vi "Camera_Focusing_updated.vi"(0 "Image Path":path=path "C:/images/img1.jpeg", 1 "CURRENT MEAN VALUE":refnum<vi>, 2 "error in":errorcluster, 3 "MEAN VALUE MAX":refnum<vi>, 4 "Filter Type":T2(ring)=enum."Differentiation", 5 "Waveform Chart":refnum<vi>, 6 "Ctl Refnum":refnum<vi>, 14 "Pattern Presence":refnum<vi>) -> (11 "Image out":T1(plugin-control), 12 "Result":bool, 13 "Reverse":bool, 15 "Mean Value Max":sgl=4.1535125 format="%.2f", 16 "error out":errorcluster, 17 "Image Dst Out":T1, 18 "Curent Mean Value":sgl=4.1535125 format="%.2f")   [LabVIEW 2019]
uses:
  <vilib>/vision/Image Controls.llb/IMAQ Image.ctl
  <vilib>/vision/NI_Vision_Development_Module.lvlib
panel:
  out "Pattern Presence":bool=TRUE
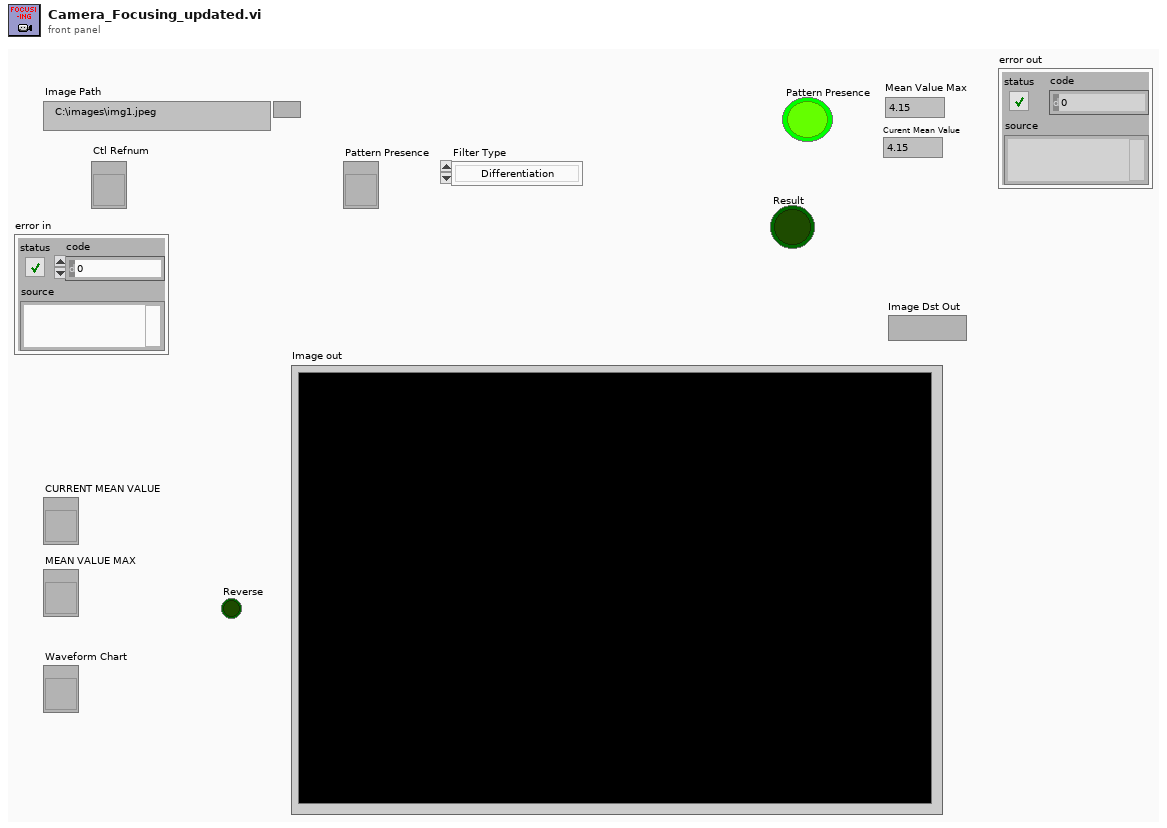
[diagram p1: front panel]
types:
  T1 = typedef "IMAQ Image.ctl" = refnum<image>
  T2 = enum16{"Convolution", "Differentiation", "Gradient", "Prewitt", "Roberts", "Sigma", "Sobel"}
  T3 = enum32{"Differentiation", "Gradient", "Prewitt", "Roberts", "Sigma", "Sobel"}
  T4 = typedef "Image Type" = u32
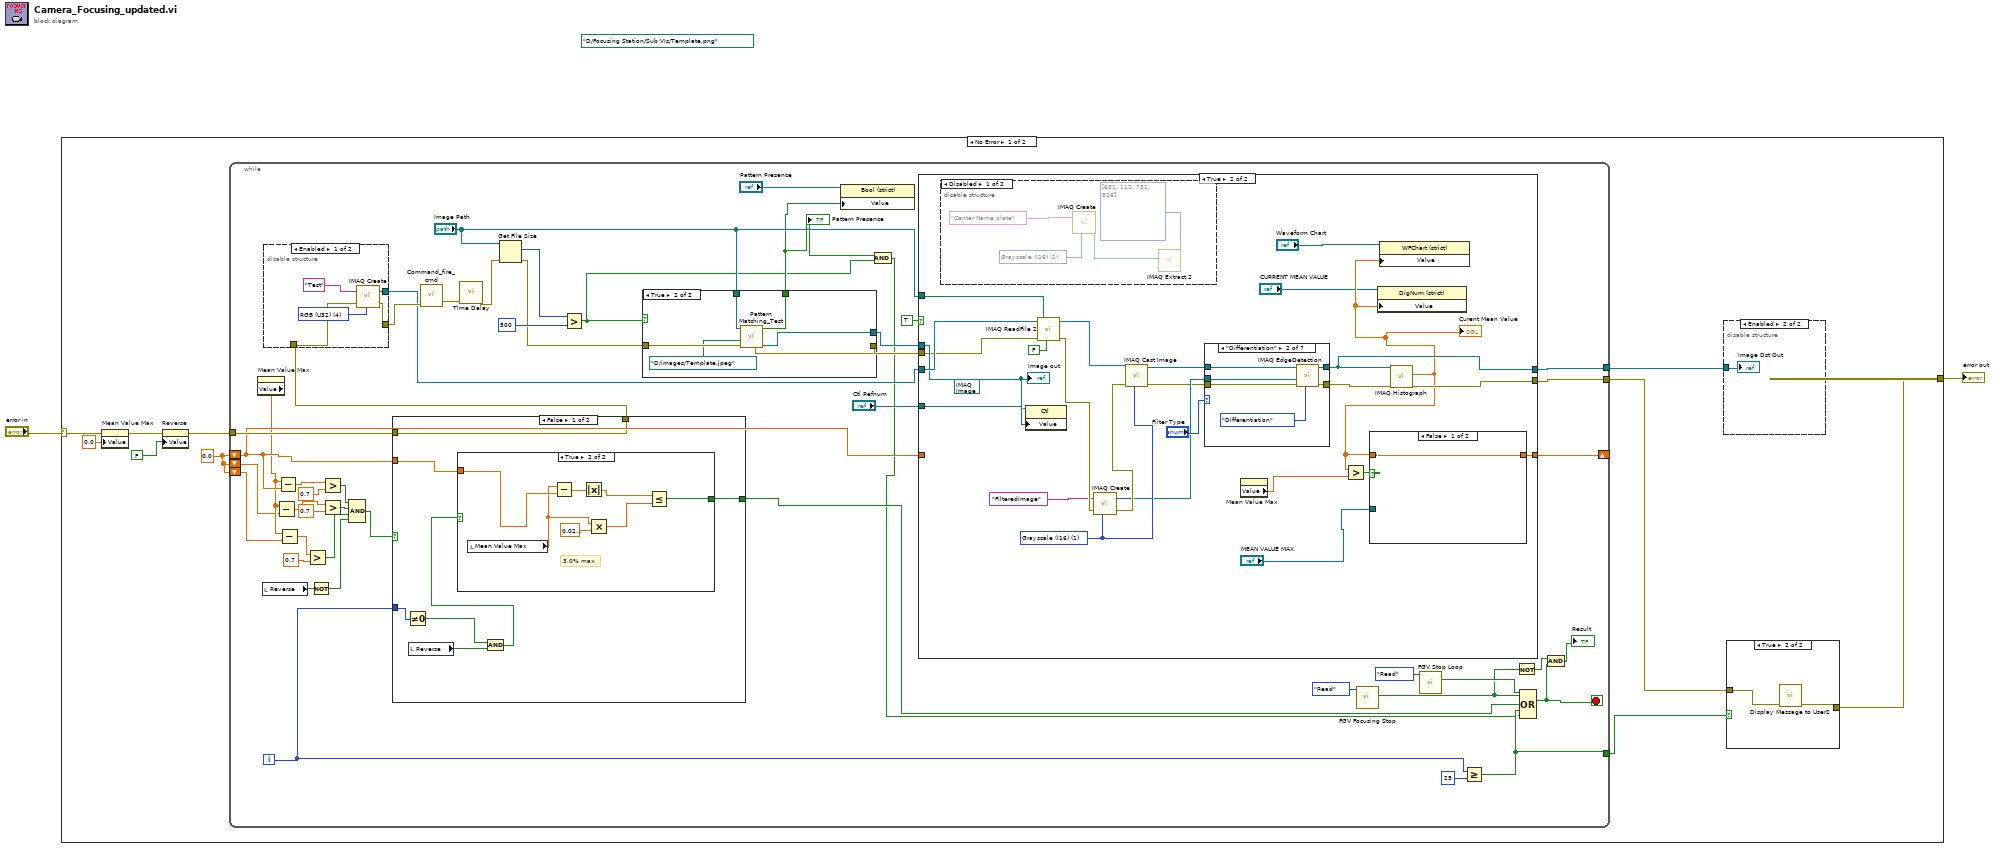
[diagram p0: block diagram]
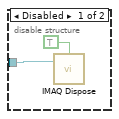
[diagram p3: hidden frame]
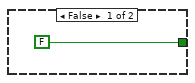
[diagram p6: hidden frame]
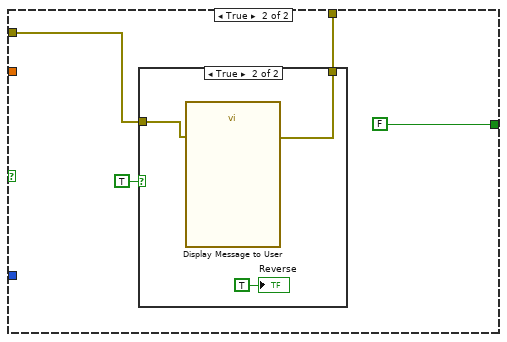
[diagram p7: hidden frame]
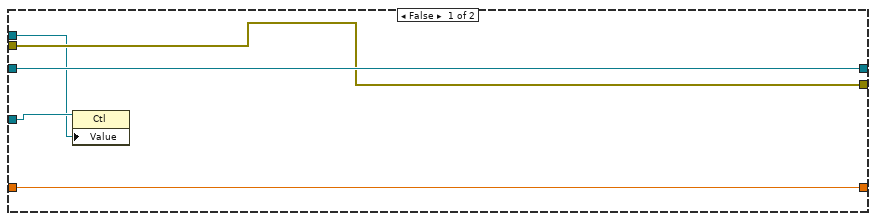
[diagram p9: hidden frame]
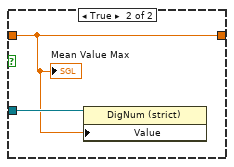
[diagram p11: hidden frame]
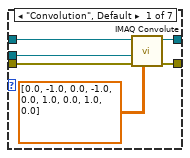
[diagram p12: hidden frame]
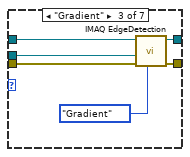
[diagram p13: hidden frame]
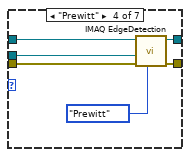
[diagram p14: hidden frame]
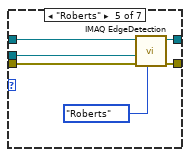
[diagram p15: hidden frame]
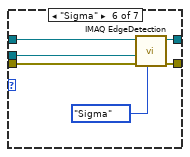
[diagram p16: hidden frame]
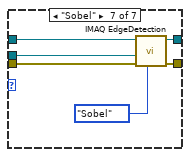
[diagram p17: hidden frame]
diagram:
  (unwired) path "D:/Focusing Station/Sub VIs/Template.png" ("Template file path")
  n1 = case shown="No Error" "error in" {
    selector: "error in" -> [w6 w181]
    tunnel: [w3 w181] -> w2
    frame No Error {
      w9 = 0.0
      n2 = property on="Mean Value Max" class="DigNum (strict)"(error in=w6, "Value"=sgl 0.0 ("Mean Value Max")) -> (error out=w8:errorcluster)  [unwired: 1 in, 1 out]
      n3 = property on="Reverse" class="Bool"(error in=w8, "Value"=FALSE ("Reverse")) -> (error out=w10:errorcluster)  [unwired: 1 in, 1 out]
      n4 = while {
        tunnel: [w66] -> w4
        tunnel: [w65] -> w12
        shift-right: [w57] -> _
        shift-left: w9 -> [w51]
        shift-left: w9 -> [w49]
        shift-left: w9 -> [w48]
        tunnel: w10 -> [w55]
        tunnel: [w30] -> w5
        i -> [w32]
        stop <- w23 stop-if-true
        n5 = property on="Mean Value Max" class="DigNum (strict)"() -> ("Value"=w50:sgl)  [unwired: 2 in, 2 out]
        n6 = local read "Reverse"() -> (w37:bool)
        n7 = Subtract(x=w50, y=w49) -> (x-y=w42:dbl)
        n8 = Subtract(x=w50, y=w51) -> (x-y=w47:dbl)
        n9 = Subtract(x=w50, y=w48) -> (x-y=w43:dbl)
        n10 = Greater?(x=w43, y=0.7) -> (0:w39:bool)
        n11 = Not(x=w37) -> (.not. x?=w36:bool)
        n12 = Greater?(x=w47, y=0.7) -> (0:w41:bool)
        n13 = Greater?(x=w42, y=0.7) -> (0:w40:bool)
        n14 = Compound Arithmetic op=AND(w41, w40, w39, w36) -> (w38:bool)
        n15 = case shown="False" w38 {
          tunnel: w32 -> [w84 _]
          tunnel: [w85 FALSE] -> w34
          tunnel: [w80 w96] -> w56
          tunnel: w55 -> [w80 w95]
          tunnel: w51 -> [w79 _]
          frame False {
            n16 = Not Equal To 0?(x=w84) -> (x != 0?=w82:bool)
            n17 = local read "Reverse"() -> (w83:bool)
            n18 = And(x=w82, y=w83) -> (x .and. y?=w81:bool)
            n19 = case shown="True" w81 {
              tunnel: [FALSE w91] -> w85
              tunnel: w79 -> [_ w88]
              frame False {
              }
              frame True {
                # "3.0% max"
                n20 = local read "Mean Value Max"() -> (w87:sgl)
                n21 = Subtract(x=w87, y=w88) -> (x-y=w93:dbl)
                n22 = Absolute Value(x=w93) -> (abs(x)=w89:dbl)
                n23 = Multiply(x=w87, y=sgl 0.03) -> (x*y=w90:sgl)
                n24 = Less Or Equal?(x=w89, y=w90) -> (x <= y?=w91:bool)
              }
            }
          }
          frame True {
            n25 = case shown="True" TRUE {
              tunnel: [w98 w100] -> w96
              tunnel: w95 -> [w98 w99]
              frame False {
              }
              frame True {
                n26 = call "Display Message to User"("error in (no error)"=w99) -> ("error out"=w100:errorcluster)  [unwired: 9 in, 1 out]
                "Reverse" <- TRUE ("Reverse")
              }
            }
          }
        }
        n27 = disable-structure shown="Enabled" {
          disable-tunnel: [w76 _] -> w61
          disable-tunnel: [w75 _] -> w60
          disable-tunnel: w56 -> [w74 _]
          frame Enabled {
            w77 = T4 4 items=["Grayscale (U8)", "Grayscale (I16)", "Grayscale (SGL)", "Complex (CSG)", "RGB (U32)", "HSL (U32)", "RGB (U64)", "Grayscale (U16)"] ("Image Type")
            n28 = call "IMAQ Create"("Image Name"="Test", "Image Type"=w77, "error in (no error)"=w74) -> ("New Image"=w75:T1, "error out"=w76:errorcluster)  [unwired: 2 in]
          }
          frame Disabled {
          }
        }
        n29 = call "Command_fire_cmd.vi"("error in"=w61) -> ("error out"=w59:errorcluster)  [unwired: 6 in, 2 out]
        n30 = call "Time Delay"("error in (no error)"=w59) -> ("error out"=w33:errorcluster)  [unwired: 10 in]
        n31 = Get File Size(file="Image Path", error in=w33) -> (size (in bytes)=w63:i64, 0:w58:errorcluster)  [unwired: 1 out]
        n32 = Greater?(x=w63, y=i64 500) -> (0:w26:bool)
        n33 = case shown="True" w26 {
          tunnel: "Image Path" -> [_ w73]
          tunnel: w58 -> [w67 w72]
          tunnel: [_ w71] -> w54
          tunnel: [_ w70] -> w27
          tunnel: [w67 w69] -> w53
          frame False {
          }
          frame True {
            n34 = call "Pattern Matching_Test.vi"("error in (no error)"=w72, "Template file path"=path "D:/images/Template.jpeg", "File Path"=w73) -> ("Image out"=w71:T1, "Pattern Presence"=w70:bool, "error out"=w69:errorcluster)  [unwired: 4 in, 2 out]
          }
        }
        "Pattern Presence" <- w27
        n35 = property class="Bool (strict)"(reference="Pattern Presence", "Value"=w27) -> ()  [unwired: 1 in, 2 out]
        n36 = And(x=w27, y=w26) -> (x .and. y?=w19:bool)
        n37 = case shown="True" TRUE {
          tunnel: "Image Path" -> [_ w130]
          tunnel: [w106 w122] -> w57
          tunnel: w51 -> [w106 _]
          tunnel: w60 -> [w105 w121]
          tunnel: [w104 w120] -> w66
          tunnel: [w105 w119] -> w65
          tunnel: w54 -> [w102 w112]
          tunnel: w53 -> [w104 w111]
          tunnel: "Ctl Refnum" -> [w103 w109]
          frame False {
            n38 = property class="Ctl"(reference=w103, "Value"=w102) -> ()  [unwired: 1 in, 2 out]
          }
          frame True {
            (unwired) T1 refnum ("New Image")
            w127 = T4 1 items=["Grayscale (U8)", "Grayscale (I16)", "Grayscale (SGL)", "Complex (CSG)", "RGB (U32)", "HSL (U32)", "RGB (U64)", "Grayscale (U16)"] ("Image Type")
            n39 = disable-structure shown="Disabled" {
              frame Disabled {
                w135 = T4 1 items=["Grayscale (U8)", "Grayscale (I16)", "Grayscale (SGL)", "Complex (CSG)", "RGB (U32)", "HSL (U32)", "RGB (U64)", "Grayscale (U16)"] ("Image Type")
                n40 = call "IMAQ Create"("Image Name"="Center Name plate", "Image Type"=w135) -> ("New Image"=w133:T1)  [unwired: 3 in, 1 out]
                n41 = call "IMAQ Extract 2"("Optional Rectangle"=i32[] [631, 112, 731, 526], "Image Dst"=w133) -> ()  [unwired: 8 in, 2 out]
              }
              frame Enabled {
              }
            }
            n42 = property class="Ctl"(reference=w109, "Value"=w112) -> ()  [unwired: 1 in, 2 out]
            n43 = call "IMAQ ReadFile 2"("Use File Path Image Type"=FALSE, "File Path"=w130, "error in (no error)"=w111, "Image"=w121) -> ("error out"=w129:errorcluster, "Image Out"=w118:T1)  [unwired: 3 in, 3 out]
            n44 = call "IMAQ Create"("Image Name"="FilteredImage", "Image Type"=w127, "error in (no error)"=w129) -> ("New Image"=w125:T1, "error out"=w128:errorcluster)  [unwired: 2 in]
            n45 = call "IMAQ Cast Image"("Image Type"=w127, "error in (no error)"=w128, "Image Src"=w118) -> ("error out"=w108:errorcluster, "Image Dst Out"=w107:T1)  [unwired: 7 in]
            n46 = case shown="\"Differentiation\"" "Filter Type" {
              tunnel: w107 -> [w143 w149 w155 w161 w167 w173 w179]
              tunnel: w108 -> [w142 w148 w154 w160 w166 w172 w178]
              tunnel: w125 -> [w141 w150 w156 w162 w168 w174 w180]
              tunnel: [w140 w145 w151 w157 w163 w169 w175] -> w124
              tunnel: [w139 w146 w152 w158 w164 w170 w176] -> w119
              frame "Convolution", Default {
                n47 = call "IMAQ Convolute"("Kernel"=sgl[][] [[0.0, -1.0, 0.0], [-1.0, 0.0, 1.0], [0.0, 1.0, 0.0]], "error in (no error)"=w142, "Image Dst"=w141, "Image Src"=w143) -> ("error out"=w140:errorcluster, "Image Dst Out"=w139:T1)  [unwired: 6 in]
              }
              frame "Differentiation" {
                n48 = call "IMAQ EdgeDetection"("Method"=T3."Differentiation", "error in (no error)"=w148, "Image Dst"=w150, "Image Src"=w149) -> ("error out"=w145:errorcluster, "Image Dst Out"=w146:T1)  [unwired: 6 in]
              }
              frame "Gradient" {
                n49 = call "IMAQ EdgeDetection"("Method"=T3."Gradient", "error in (no error)"=w154, "Image Dst"=w156, "Image Src"=w155) -> ("error out"=w151:errorcluster, "Image Dst Out"=w152:T1)  [unwired: 6 in]
              }
              frame "Prewitt" {
                n50 = call "IMAQ EdgeDetection"("Method"=T3."Prewitt", "error in (no error)"=w160, "Image Dst"=w162, "Image Src"=w161) -> ("error out"=w157:errorcluster, "Image Dst Out"=w158:T1)  [unwired: 6 in]
              }
              frame "Roberts" {
                n51 = call "IMAQ EdgeDetection"("Method"=T3."Roberts", "error in (no error)"=w166, "Image Dst"=w168, "Image Src"=w167) -> ("error out"=w163:errorcluster, "Image Dst Out"=w164:T1)  [unwired: 6 in]
              }
              frame "Sigma" {
                n52 = call "IMAQ EdgeDetection"("Method"=T3."Sigma", "error in (no error)"=w172, "Image Dst"=w174, "Image Src"=w173) -> ("error out"=w169:errorcluster, "Image Dst Out"=w170:T1)  [unwired: 6 in]
              }
              frame "Sobel" {
                n53 = call "IMAQ EdgeDetection"("Method"=T3."Sobel", "error in (no error)"=w178, "Image Dst"=w180, "Image Src"=w179) -> ("error out"=w175:errorcluster, "Image Dst Out"=w176:T1)  [unwired: 6 in]
              }
            }
            n54 = property on="Mean Value Max" class="DigNum (strict)"() -> ("Value"=w113:sgl)  [unwired: 2 in, 2 out]
            n55 = call "IMAQ Histograph"("error in (no error)"=w124, "Image"=w119) -> ("error out"=w120:errorcluster, "Mean Value"=w117:sgl)  [unwired: 6 in, 2 out]
            "Curent Mean Value" <- w117
            n56 = Greater?(x=w117, y=w113) -> (0:w123:bool)
            n57 = case shown="False" w123 {
              tunnel: w117 -> [w136 w137]
              tunnel: [w136 w137] -> w122
              tunnel: "MEAN VALUE MAX" -> [_ w138]
              frame False {
              }
              frame True {
                n58 = property class="DigNum (strict)"(reference=w138, "Value"=w137) -> ()  [unwired: 1 in, 2 out]
                "Mean Value Max" <- w137
              }
            }
            n59 = property class="DigNum (strict)"(reference="CURRENT MEAN VALUE", "Value"=w117) -> ()  [unwired: 1 in, 2 out]
            n60 = property class="WFChart (strict)"(reference="Waveform Chart", "Value"=w117) -> ()  [unwired: 1 in, 2 out]
            "Image out" <- w112
          }
        }
        n61 = call "FGV Focusing Stop.vi"("Action"=enum16{"Initialize", "Read", "Write"}."Read") -> ("Out"=w21:bool)  [unwired: 9 in, 1 out]
        n62 = call "FGV Stop Loop.vi"("Action"=enum16{"Initialize", "Read", "Write"}."Read") -> ("Out"=w28:bool)  [unwired: 9 in, 1 out]
        n63 = Greater Or Equal?(x=w32, y=25) -> (x >= y?=w30:bool)
        n64 = Not(x=w21) -> (.not. x?=w22:bool)
        n65 = Compound Arithmetic op=OR(w28, w21, w34, w30, w19) -> (w23:bool)
        n66 = And(x=w22, y=w23) -> (x .and. y?=→"Result":bool)
      }
      n67 = disable-structure shown="Enabled" {
        disable-tunnel: w12 -> [w17 w18]
        frame Disabled {
          n68 = call "IMAQ Dispose"("All Images? (No)"=TRUE, "Image"=w17) -> ()  [unwired: 4 in, 1 out]
        }
        frame Enabled {
          "Image Dst Out" <- w18
        }
      }
      n69 = case shown="True" w5 {
        tunnel: w4 -> [w13 w15]
        tunnel: [w13 w14] -> w3
        frame False {
        }
        frame True {
          n70 = call "Display Message to User2"("error in (no error)"=w15) -> ("error out"=w14:errorcluster)  [unwired: 9 in, 1 out]
        }
      }
    }
    frame Error {
    }
  }
  "error out" <- w2
